vi "SVI_NewE2E_SerialSendReceive.vi"(5 "NAK":string="N", 6 "End Char":string="\n", 7 "ACK":string="A", 8 "error in (no error)":errorcluster, 9 "Command":string, 10 "Message Type":enum16{"Expecting Response", "Expecting ACK"}(ring), 11 "VISA Refnum in":refnum<visa-resource-name>) -> (0 "error out":errorcluster, 1 "Attempt":i32, 2 "Received":string, 3 "VISA resource name out":refnum<visa-resource-name>)   [LabVIEW 2014]
panel:
  out "Array":string[](array[string])
  in  "Wait Time (ms)":u32=10
  out "Attempt time":u32
  in  "Retries":i32=50
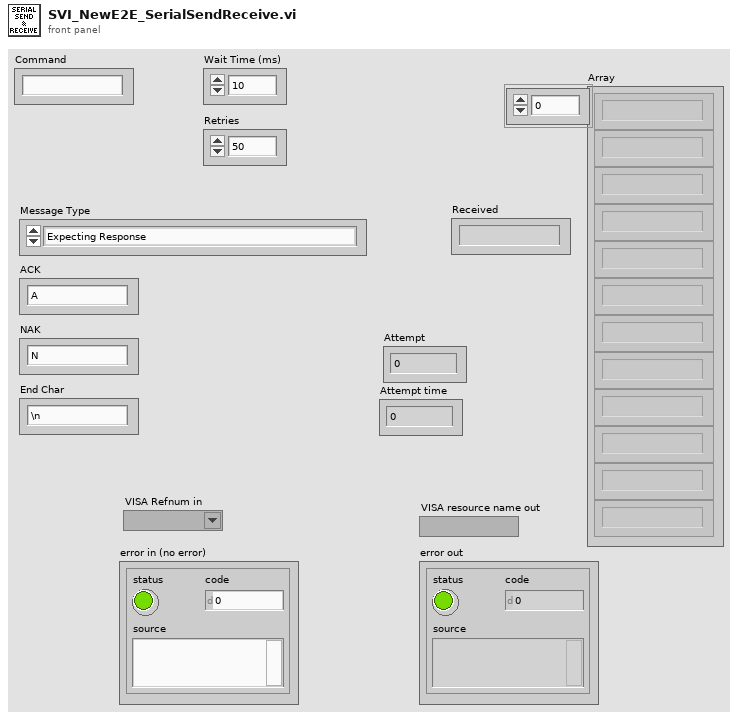
[diagram p1: front panel]
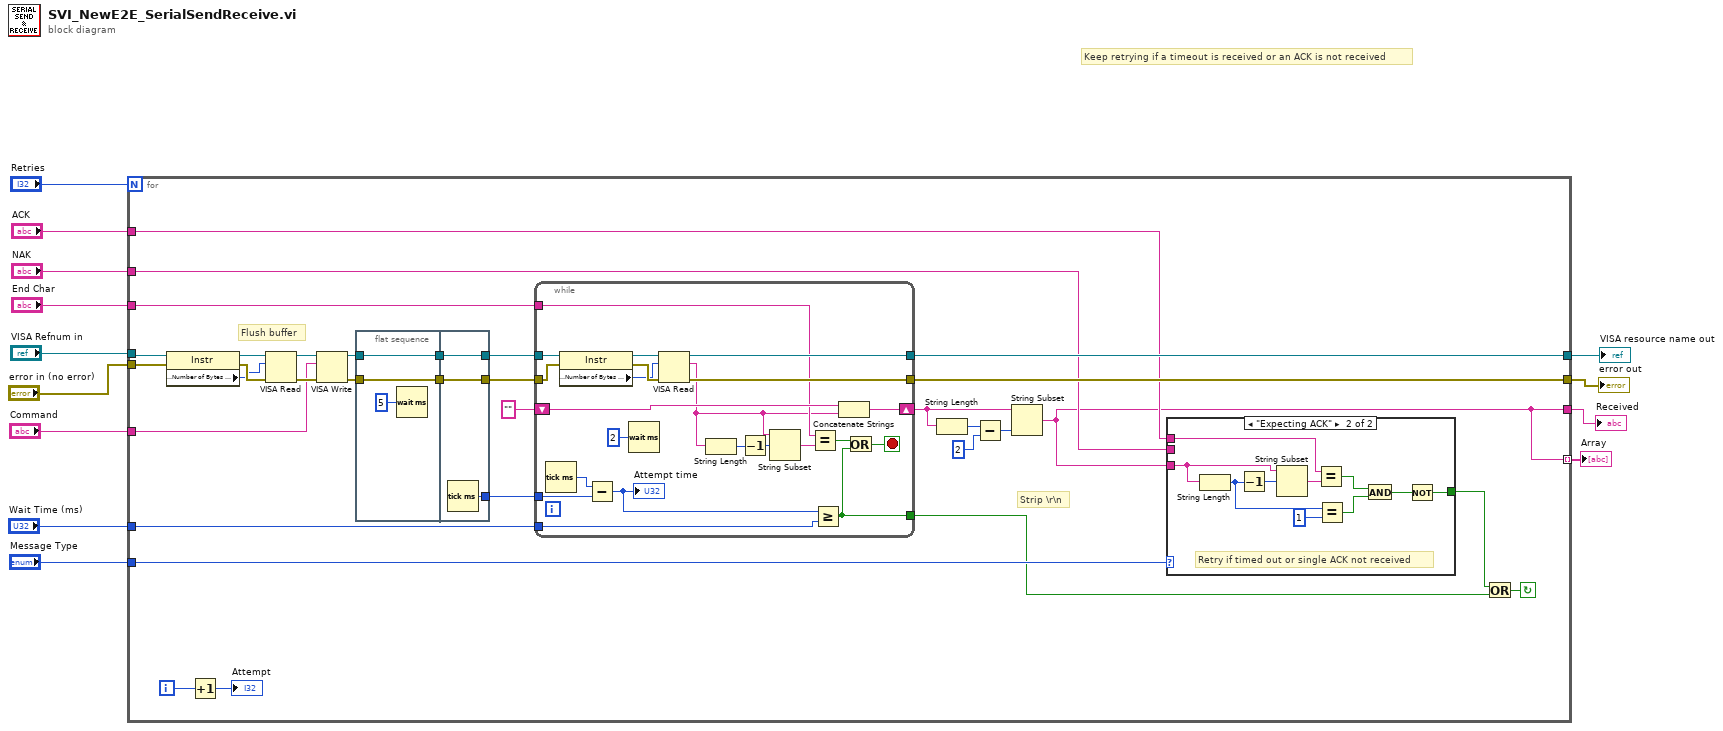
[diagram p0: block diagram]
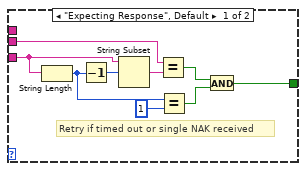
[diagram p2: hidden frame]
diagram:
  # "Keep retrying if a timeout is received or an ACK is not received"
  n1 = for {
    N: "Retries" -> [_]
    tunnel: "error in (no error)" -> [w39]
    tunnel: "VISA Refnum in" -> [w38]
    tunnel: "Wait Time (ms)" -> [w34]
    tunnel: [w33] -> w7
    tunnel: [w32] -> w9
    tunnel: [w17] -> w8
    tunnel: "End Char" -> [w26]
    tunnel: "NAK" -> [w23]
    tunnel: "Command" -> [w25]
    tunnel: "Message Type" -> [w24]
    tunnel: "ACK" -> [w19]
    tunnel: [w17] -> w1 mode=indexing
    i -> [w31]
    stop <- w22 continue-if-true
    # "Strip \\r\\n"
    # "Flush buffer"
    n2 = property class="Instr"(reference=w38, error in=w39) -> (reference out=w44:refnum<visa-resource-name>, error out=w43:errorcluster, "Serial Settings:Number of Bytes at Serial Port"=w42:u32)
    n3 = Increment(x=w31) -> (x+1=→"Attempt":i32)
    n4 = VISA Read(VISA resource name=w44, byte count=w42, error in (no error)=w43) -> (VISA resource name out=w41:refnum<visa-resource-name>, error out=w40:errorcluster)  [unwired: 2 out]
    n5 = VISA Write(VISA resource name=w41, write buffer=w25, error in (no error)=w40) -> (VISA resource name out=w45:refnum<visa-resource-name>, error out=w46:errorcluster)  [unwired: 1 out]
    n6 = flat-sequence {
      tunnel: w46 -> [w90]
      tunnel: w45 -> [w89]
      tunnel: [w90] -> w30
      tunnel: [w89] -> w29
      tunnel: [w92] -> w35
      tunnel: [w93] -> w36
      tunnel: w30 -> [w93]
      tunnel: w29 -> [w92]
      tunnel: [w91] -> w28
      frame #0 {
        n7 = Wait (ms)(milliseconds to wait=u32 5) -> ()  [unwired: 1 out]
      }
      frame #1 {
        n8 = Tick Count (ms)() -> (millisecond timer value=w91:u32)
      }
    }
    n9 = while {
      tunnel: w35 -> [w85]
      tunnel: [w83] -> w32
      shift-right: [w76] -> w18
      shift-left: "" -> [w81]
      tunnel: w28 -> [w79]
      tunnel: w36 -> [w84]
      tunnel: [w82] -> w33
      tunnel: w34 -> [w78]
      tunnel: w26 -> [w70]
      tunnel: [w67] -> w20
      stop <- w69 stop-if-true
      n10 = Tick Count (ms)() -> (millisecond timer value=w80:u32)
      n11 = property class="Instr"(reference=w85, error in=w84) -> (reference out=w87:refnum<visa-resource-name>, error out=w86:errorcluster, "Serial Settings:Number of Bytes at Serial Port"=w77:u32)
      n12 = Subtract(x=w80, y=w79) -> (x-y=w75:u32)
      "Attempt time" <- w75
      n13 = Wait (ms)(milliseconds to wait=u32 2) -> ()  [unwired: 1 out]
      n14 = VISA Read(VISA resource name=w87, byte count=w77, error in (no error)=w86) -> (VISA resource name out=w83:refnum<visa-resource-name>, read buffer=w66:string, error out=w82:errorcluster)  [unwired: 1 out]
      n15 = String Length(string=w66) -> (length=w73:i32)
      n16 = Decrement(x=w73) -> (x-1=w72:i32)
      n17 = String Subset(string=w66, offset (0)=w72) -> (substring=w71:string)  [unwired: 1 in]
      n18 = Equal?(x=w70, y=w71) -> (x = y?=w68:bool)
      n19 = Greater Or Equal?(x=w75, y=w78) -> (x >= y?=w67:bool)
      n20 = Concatenate Strings(w81, w66) -> (w76:string)
      n21 = Or(x=w68, y=w67) -> (x .or. y?=w69:bool)
    }
    n22 = String Length(string=w18) -> (length=w15:i32)
    n23 = Subtract(x=w15, y=2) -> (x-y=w16:i32)
    n24 = String Subset(string=w18, length (rest)=w16) -> (substring=w17:string)  [unwired: 1 in]
    n25 = case shown="\"Expecting ACK\"" w24 {
      tunnel: [w47 w56] -> w21
      tunnel: w23 -> [w53 _]
      tunnel: w17 -> [w52 w57]
      tunnel: w19 -> [_ w58]
      frame "Expecting Response", Default {
        # "Retry if timed out or single NAK received"
        n26 = String Length(string=w52) -> (length=w49:i32)
        n27 = Decrement(x=w49) -> (x-1=w55:i32)
        n28 = String Subset(string=w52, offset (0)=w55) -> (substring=w54:string)  [unwired: 1 in]
        n29 = Equal?(x=w53, y=w54) -> (x = y?=w51:bool)
        n30 = Equal?(x=w49, y=1) -> (x = y?=w50:bool)
        n31 = And(x=w51, y=w50) -> (x .and. y?=w47:bool)
      }
      frame "Expecting ACK" {
        # "Retry if timed out or single ACK not received"
        n32 = String Length(string=w57) -> (length=w64:i32)
        n33 = Decrement(x=w64) -> (x-1=w60:i32)
        n34 = String Subset(string=w57, offset (0)=w60) -> (substring=w61:string)  [unwired: 1 in]
        n35 = Equal?(x=w58, y=w61) -> (x = y?=w62:bool)
        n36 = Equal?(x=w64, y=1) -> (x = y?=w63:bool)
        n37 = And(x=w62, y=w63) -> (x .and. y?=w59:bool)
        n38 = Not(x=w59) -> (.not. x?=w56:bool)
      }
    }
    n39 = Or(x=w21, y=w20) -> (x .or. y?=w22:bool)
  }
  "error out" <- w7
  "VISA resource name out" <- w9
  "Received" <- w8
  "Array" <- w1
